vi "Write Holding Regs.vi"(0 "reference in":refnum<class "MB_MODULE.lvclass">, 5 "starting address":u16, 7 "Regs":u16[](array[numeric]), 11 "error in (no error)":errorcluster) -> (4 "reference out":refnum<class "MB_MODULE.lvclass">, 15 "error out":errorcluster)   [LabVIEW 2019, in "MB_MODULE.lvclass"]
uses:
  MB_MODULE.lvclass
  MB_MODULE.lvclass/MB_MODULE.ctl
  <vilib>/NI/Modbus Library/API/Master/Modbus Master.lvclass
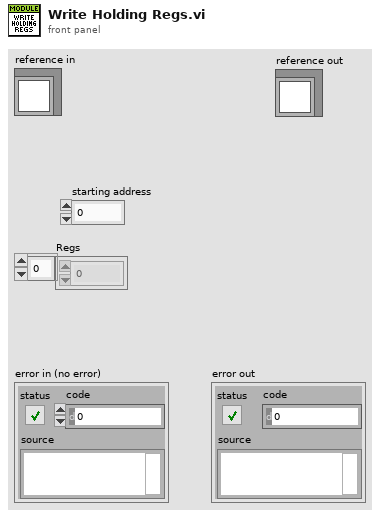
[diagram p1: front panel]
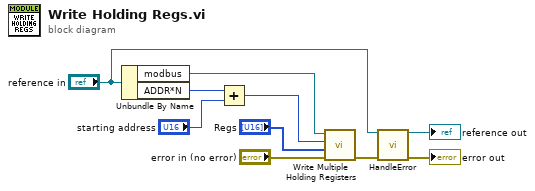
[diagram p0: block diagram]
diagram:
  n1 = Unbundle By Name("reference in") -> ("modbus"=w5:refnum<class "Modbus Master.lvclass">, "ADDR*N"=w6:u16)
  n2 = Add(x=w6, y="starting address") -> (x+y=w8:u16)
  n3 = call-dynamic "Write Multiple Holding Registers.vi"("error in"="error in (no error)", "registers to write"="Regs", "starting address"=w8, "Modbus master in"=w5) -> ("error out"=w4:errorcluster)  [unwired: 6 in, 1 out]
  n4 = call "HandleError.vi"("reference in"="reference in", "error in (no error)"=w4) -> ("reference out"=→"reference out":refnum<class "MB_MODULE.lvclass">, "error out"=→"error out":errorcluster)  [unwired: 12 in]
